vi "Load States.vi"(8 "Error In":errorcluster, 10 "States Nodes":refnum<k20>[](array[refnum]), 11 "UIPs":string[](array[string])) -> (0 "Error Out":errorcluster, 3 "States Variant":variant)   [LabVIEW 2020, in "UIM.lvlib" / "UIM.lvclass"]
uses:
  UIM.lvclass
  UIP Interface/UIP Interface.lvclass
  <vilib>/xml/Close Reference(Node).vi
  UIM.lvclass/UIM.ctl
  <resource>/objmgr/DOMUserDefRef.rc
  <vilib>/xml/NI_XML.lvlib
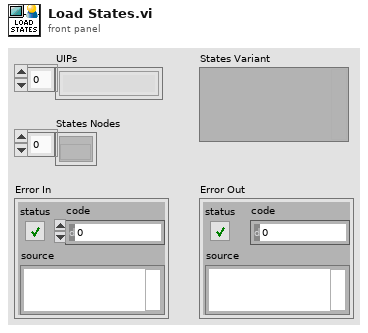
[diagram p1: front panel]
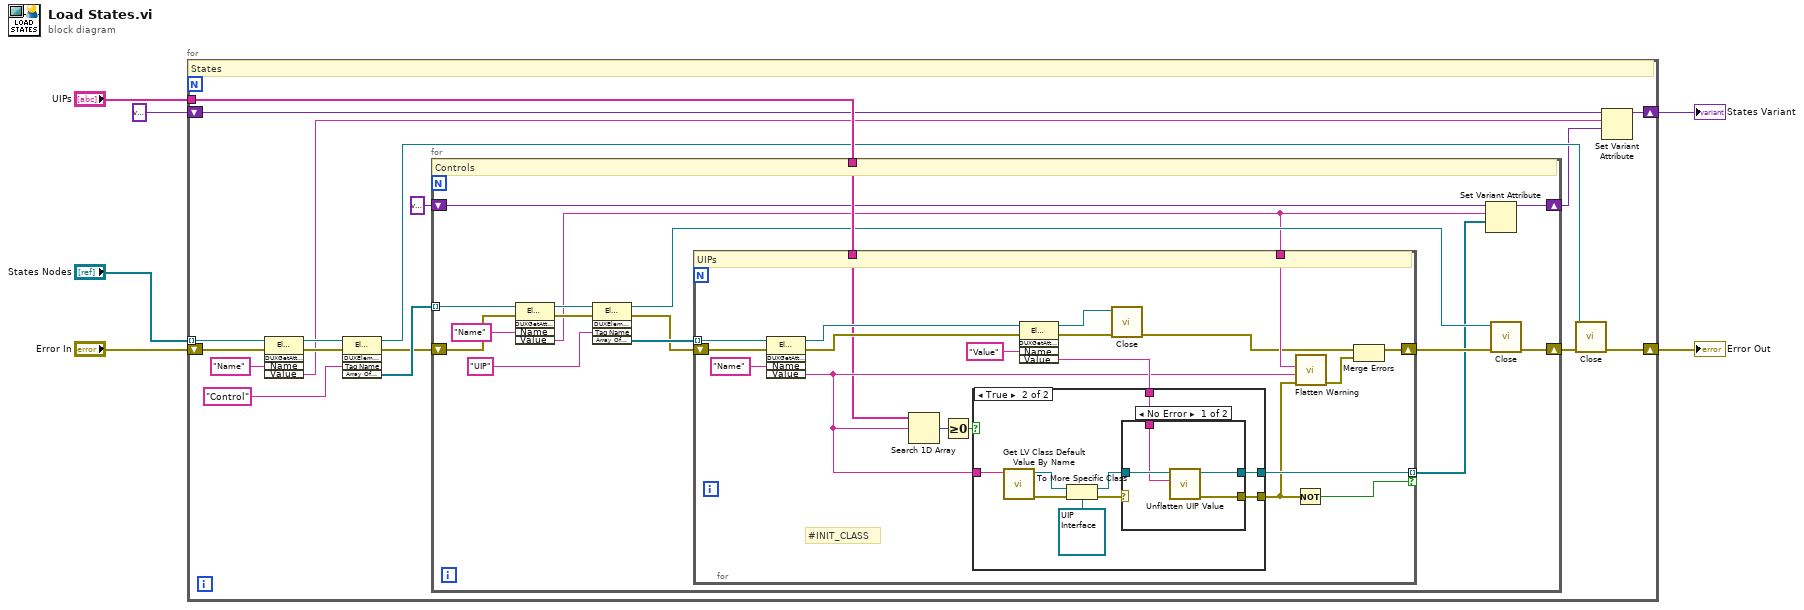
[diagram p0: block diagram]
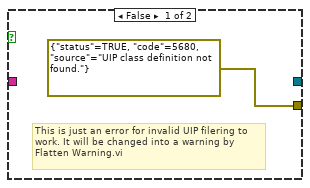
[diagram p2: hidden frame]
diagram:
  n1 = for {
    tunnel: "States Nodes" -> [w23] mode=indexing
    shift-right: [w9] -> w2
    shift-left: variant -> [w10]
    shift-right: [w14] -> w3
    shift-left: "Error In" -> [w18]
    tunnel: "UIPs" -> [w17]
    # "States"
    n2 = invoke class="Element" method="DUXGetAttribute"(reference=w23, error in=w18, "Name"="Name") -> (reference out=w21:refnum<k20>, error out=w13:errorcluster, "Value"=w7:string)  [unwired: 2 in, 2 out]
    n3 = invoke class="Element" method="DUXElementGetElementsByTagNameArray"(reference=w21, error in=w13, "Tag Name"="Control") -> (reference out=w15:refnum<k20>, error out=w12:errorcluster, "Array Of Elements"=w19:refnum<k20>[])  [unwired: 2 in, 2 out]
    n4 = for {
      tunnel: w19 -> [w39] mode=indexing
      shift-right: [w30] -> w16
      shift-left: w12 -> [w34]
      tunnel: w17 -> [w31]
      shift-right: [w24] -> w8
      shift-left: variant -> [w27]
      # "Controls"
      n5 = invoke class="Element" method="DUXGetAttribute"(reference=w39, error in=w34, "Name"="Name") -> (reference out=w37:refnum<k20>, error out=w33:errorcluster, "Value"=w26:string)  [unwired: 2 in, 2 out]
      n6 = invoke class="Element" method="DUXElementGetElementsByTagNameArray"(reference=w37, error in=w33, "Tag Name"="UIP") -> (reference out=w29:refnum<k20>, error out=w32:errorcluster, "Array Of Elements"=w35:refnum<k20>[])  [unwired: 2 in, 2 out]
      n7 = for {
        tunnel: w35 -> [w59] mode=indexing
        tunnel: w26 -> [w52]
        tunnel: [w50] -> w25 mode=indexing if=w48
        shift-right: [w47] -> w28
        shift-left: w32 -> [w55]
        tunnel: w31 -> [w40]
        # "#INIT_CLASS"
        # "UIPs"
        n8 = invoke class="Element" method="DUXGetAttribute"(reference=w59, error in=w55, "Name"="Name") -> (reference out=w58:refnum<k20>, error out=w54:errorcluster, "Value"=w51:string)  [unwired: 2 in, 2 out]
        n9 = Search 1D Array(1D array=w40, element=w51) -> (index of element=w42:i32)  [unwired: 1 in]
        n10 = Greater Or Equal To 0?(x=w42) -> (x >= 0?=w41:bool)
        n11 = invoke class="Element" method="DUXGetAttribute"(reference=w58, error in=w54, "Name"="Value") -> (reference out=w44:refnum<k20>, error out=w45:errorcluster, "Value"=w53:string)  [unwired: 2 in, 2 out]
        n12 = case shown="True" w41 {
          tunnel: w53 -> [_ w64]
          tunnel: [_ w63] -> w50
          tunnel: [errorcluster {"status"=TRUE, "code"=5680, "source"="UIP class definition not found."} ("error constant") w62] -> w49
          tunnel: w51 -> [_ w61]
          frame False {
            # "This is just an error for invalid UIP filering to\nwork. It will be changed into a warning by\nFlatten Warning.vi"
          }
          frame True {
            n13 = call <vilib>:"Get LV Class Default Value By Name.vi"("class name"=w61) -> ("error out"=w68:errorcluster, "object"=w69:refnum<class>)  [unwired: 9 in]
            n14 = To More Specific Class(target class=refnum<class "UIP Interface.lvclass"> refnum ("UIMLib.lvlib:UIP Interface.lvclass"), reference=w69, error in=w68) -> (specific class reference=w65:refnum<class "UIP Interface.lvclass">, error out=w66:errorcluster)
            n15 = case shown="No Error" w66 {
              selector: w66 -> [_ w74]
              tunnel: w65 -> [w73 _]
              tunnel: w64 -> [w72 _]
              tunnel: [w71 w74] -> w62
              tunnel: [w70 _] -> w63
              frame No Error {
                n16 = call-dynamic "Unflatten UIP Value.vi"("String Value"=w72, "UIP In"=w73) -> ("Error Out"=w71:errorcluster, "UIP Out"=w70:refnum<class "UIP Interface.lvclass">)  [unwired: 8 in]
              }
              frame Error {
              }
            }
          }
        }
        n17 = call-poly <vilib>:"Close.vi"("error in (no error)"=w45, "node"=w44) -> ("error out"=w43:errorcluster)  [unwired: 7 in]
        n18 = Not(x=w49) -> (.not. x?=w48:bool)
        n19 = call "Flatten Warning.vi"("Error In"=w49, "UIP Name"=w51, "Label.Text"=w52) -> ("Error Out"=w46:errorcluster)  [unwired: 8 in]
        n20 = Merge Errors(w43, w46) -> (w47:errorcluster)
      }
      n21 = Set Variant Attribute(Variant=w27, name=w26, value=w25) -> (Variant out=w24:variant)  [unwired: 1 in, 2 out]
      n22 = call-poly <vilib>:"Close.vi"("error in (no error)"=w28, "node"=w29) -> ("error out"=w30:errorcluster)  [unwired: 7 in]
    }
    n23 = call-poly <vilib>:"Close.vi"("error in (no error)"=w16, "node"=w15) -> ("error out"=w14:errorcluster)  [unwired: 7 in]
    n24 = Set Variant Attribute(Variant=w10, name=w7, value=w8) -> (Variant out=w9:variant)  [unwired: 1 in, 2 out]
  }
  "Error Out" <- w3
  "States Variant" <- w2
